vi "FTW-Supervisor-Shutdown.vi"(0 "FTW Supervisor Connection":refnum<class "FTW-Supervisor-Connector.lvclass">, 11 "error in":errorcluster) -> (15 "error out":errorcluster)   [LabVIEW 2014, in "FTW-Supervisor.lvclass"]
uses:
  FTW-Supervisor.lvclass
  connector/FTW-Supervisor-Connector.lvclass
panel:
  in  "Timeout":i32=5000 format="%dmsec"
  # "Inputs"
  # "Outputs"
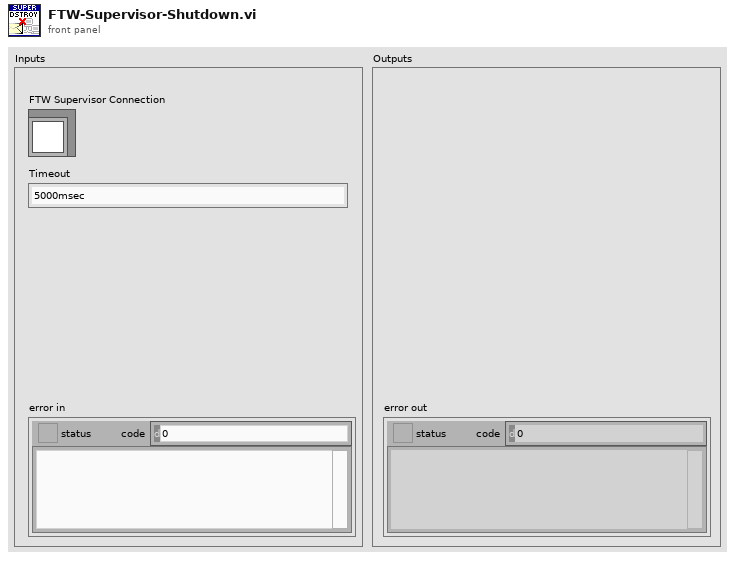
[diagram p1: front panel]
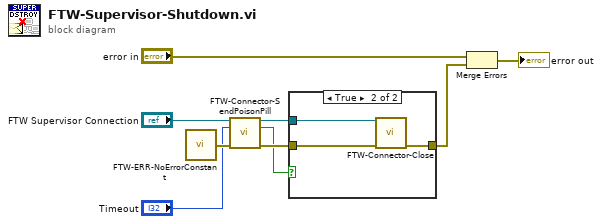
[diagram p0: block diagram]
diagram:
  n1 = call "FTW-ERR-NoErrorConstant.vi"() -> ("no error"=w3:errorcluster)
  n2 = call-dynamic "FTW-Connector-SendPoisonPill.vi"("FTW Actor Connector"="FTW Supervisor Connection", "Timeout"="Timeout", "error in"=w3) -> ("FTW Actor Connector out"=w7:refnum<class "FTW-Supervisor-Connector.lvclass">, "Shutting Down?"=w1:bool, "error out"=w6:errorcluster)  [unwired: 9 in, 1 out]
  n3 = case shown="True" w1 {
    tunnel: w7 -> [_ w13]
    tunnel: w6 -> [w10 w12]
    tunnel: [w10 w11] -> w4
    frame False {
    }
    frame True {
      n4 = call-dynamic "FTW-Connector-Close.vi"("FTW Actor Connector"=w13, "error in"=w12) -> ("error out"=w11:errorcluster)  [unwired: 13 in]
    }
  }
  n5 = Merge Errors("error in", w4) -> (→"error out":errorcluster)
